vi "Read Elevator Command.vi"(6 "Reset Idle State":bool, 8 "Button Cluster":T3, 9 "Axes":dbl[](array[numeric]), 10 "Driver Buttons":bool[](array[boolean]), 11 "Call Context":T1) -> (0 "Idle Mode":T2, 3 "Command":T4)   [LabVIEW 2014]
uses:
  Elevator Command.ctl
  Common Code/Elevator Idle Mode.ctl
  Real-Life Controls/Button Cluster.ctl
  <vilib>/Rock Robotics/WPI/DriverStation/WPI_DriverStationDerivedRobotMode.ctl
  Common Code/Elevator State.ctl
  Common Code/Change Detect.vi
  Common Code/Change Detect Boolean.vi
  Robot Global Data.vi
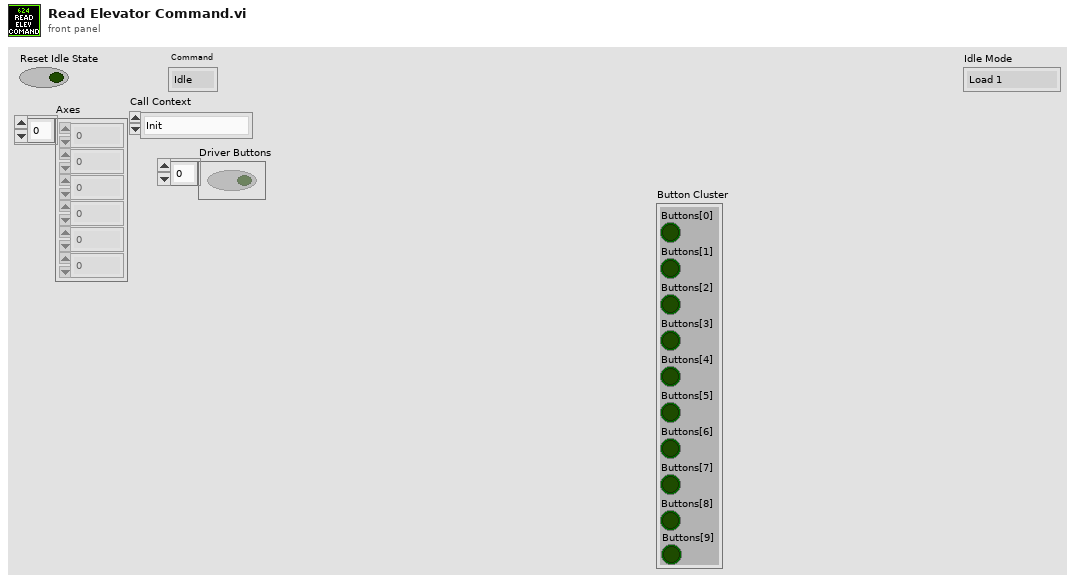
[diagram p1: front panel]
types:
  T1 = typedef "WPI_DriverStationDerivedRobotMode.ctl" = enum16{"Init", "Execute", "Stop"}
  T2 = typedef "Elevator Idle Mode.ctl" = enum16{"Load 1", "Load 2", "Load 3", "Load Can", "Untip Can", "Step Load", "Drop Stack", "Raw Height"}
  T3 = typedef "Button Cluster.ctl" = cluster{"Buttons[0]":bool, "Buttons[1]":bool, "Buttons[2]":bool, "Buttons[3]":bool, "Buttons[4]":bool, "Buttons[5]":bool, "Buttons[6]":bool, "Buttons[7]":bool, "Buttons[8]":bool, "Buttons[9]":bool}
  T4 = typedef "Elevator Command.ctl" = enum16{"Idle", "Load 1", "Load 2", "Load 3", "Drop Stack", "Eject Stack", "Untip Trashcan", "Load Trashcan", "HP Load", "HP Score"}
  T5 = typedef "Elevator State.ctl" = enum16{"Idle", "Goto Load Position", "Wait for Load", "Load Drop", "Load Lift", "Drop Stack", "Goto Eject Position", "Eject ", "Raise Trashcan", "Open Stabilizer", "Untip Drop", "Untip Wait", "Untip Lift", "Abort Load", "HP Load Wait", "HP Load Drop", "HP Load Lift", "HP Load Abort", "Close Stabilizer", "HP Load Unfinish", "HP Load Score", "HP Load Finish", "HP Goto Finish Down", "HP Goto Finish Up", "Full"}
  T6 = typedef "Elevator Status.ctl" = cluster{"Height":dbl, "Enc Value":dbl, "Limit Override":bool, "Mode":T7, "High IR":bool, "Motor Out":dbl, "Ping Detect":bool, "Auto Elevator Indicators":T8, "Master Current":dbl, "Slave Current":dbl, "High Current":bool, "Current Tripped":bool, "Top Limit":bool, "Bottom Limit":bool, "Eject Piston":bool, "Stabilizer":bool, "Finger":bool, "Finger Height":dbl, "Finger Raw":dbl, "Finger at Bottom":bool}
  T7 = typedef "Elevator Mode.ctl" = enum16{"Manual", "Safe", "Auto"}
  T8 = typedef "Auto Elevator Indicators.ctl" = cluster{"Target Out":dbl, "Storing Trashcan?":bool, "State":T5, "In Range":bool, "Store Can Command":bool, "HP Load":bool}
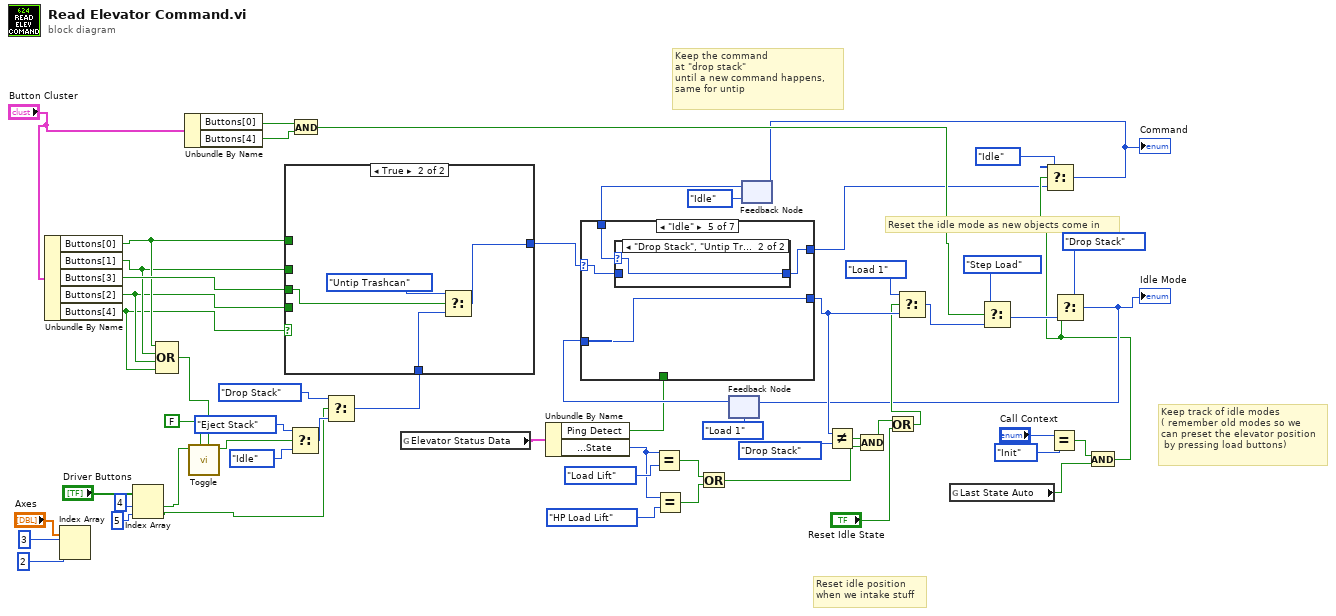
[diagram p0: block diagram]
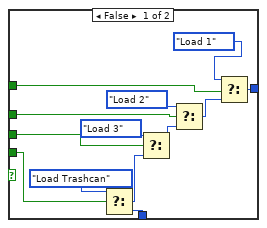
[diagram p2: hidden frame]
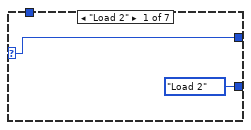
[diagram p3: hidden frame]
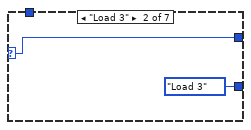
[diagram p4: hidden frame]
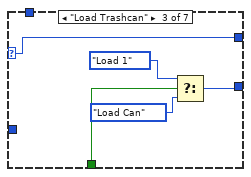
[diagram p5: hidden frame]
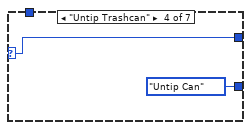
[diagram p6: hidden frame]
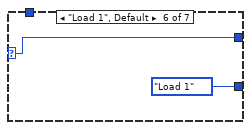
[diagram p8: hidden frame]
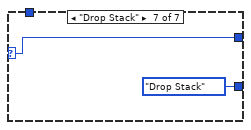
[diagram p9: hidden frame]
diagram:
  # "Keep the command\nat \"drop stack\"\nuntil a new command happens,\nsame for untip"
  # "Reset idle position\nwhen we intake stuff"
  # "Keep track of idle modes\n( remember old modes so we\ncan preset the elevator position\n by pressing load buttons)"
  # "Reset the idle mode as new objects come in"
  n1 = Unbundle By Name("Button Cluster") -> ("Buttons[0]"=w19:bool, "Buttons[1]"=w18:bool, "Buttons[3]"=w32:bool, "Buttons[2]"=w17:bool, "Buttons[4]"=w16:bool)
  n2 = Index Array(array="Axes", index #1=3 ("index"), index #2=2 ("index")) -> ()  [unwired: 2 out]
  n3 = Index Array(array="Driver Buttons", index #1=4 ("index"), index #2=5 ("index")) -> (element #1=w10:bool, element #2=w6:bool)
  n4 = Compound Arithmetic op=OR(w19, w18, w17, w16) -> (w15:bool)
  n5 = Unbundle By Name("Button Cluster") -> ("Buttons[0]"=w44:bool, "Buttons[4]"=w43:bool)
  n6 = call "Toggle.vi"("Reinit?"=w15, "Initial Value"=FALSE, "In"=w10) -> ("Toggled"=w20:bool)  [unwired: 8 in]
  n7 = Select(t=Elevator_Command."Eject Stack", s=w20, f=Elevator_Command."Idle" ("t")) -> (s? t:f=w56:T4)
  n8 = And(x=w44, y=w43) -> (x .and. y?=w42:bool)
  n9 = Select(t=Elevator_Command."Drop Stack", s=w6, f=w56) -> (s? t:f=w33:T4)
  n10 = case shown="True" w16 {
    tunnel: w33 -> [w64 w74]
    tunnel: [w63 w73] -> w49
    tunnel: w19 -> [w62 _]
    tunnel: w18 -> [w61 _]
    tunnel: w32 -> [w60 w72]
    tunnel: w17 -> [w59 _]
    frame False {
      n11 = Select(t=Elevator_Command."Load Trashcan", s=w59, f=w64) -> (s? t:f=w70:T4)
      n12 = Select(t=Elevator_Command."Load 3", s=w60, f=w70) -> (s? t:f=w66:T4)
      n13 = Select(t=Elevator_Command."Load 2", s=w61, f=w66) -> (s? t:f=w65:T4)
      n14 = Select(t=Elevator_Command."Load 1", s=w62, f=w65) -> (s? t:f=w63:T4)
    }
    frame True {
      n15 = Select(t=Elevator_Command."Untip Trashcan", s=w72, f=w74) -> (s? t:f=w73:T4)
    }
  }
  n16 = global read "Robot Global Data.vi" "Elevator Status Data"() -> (w31:T6)
  n17 = Unbundle By Name(w31) -> ("Ping Detect"=w21:bool, "Auto Elevator Indicators.State"=w28:T5)
  n18 = Equal?(x=w28, y=Elevator_State."Load Lift") -> (x = y?=w27:bool)
  n19 = Equal?(x=w28, y=Elevator_State."HP Load Lift") -> (x = y?=w25:bool)
  n20 = Or(x=w27, y=w25) -> (x .or. y?=w26:bool)
  n21 = feedback #1(Elevator_Idle_Mode."Load 1" ("Idle Mode")) -> (w48:T2)
  n22 = feedback #2(Elevator_Command."Idle" ("t")) -> (w36:T4)
  n23 = case shown="\"Idle\"" w49 {
    selector: w49 -> [w76 w78 w84 w85 w88 w93 w95]
    tunnel: [Elevator_Idle_Mode."Load 2" ("Idle Mode") Elevator_Idle_Mode."Load 3" ("Idle Mode") w80 Elevator_Idle_Mode."Untip Can" ("Idle Mode") w90 Elevator_Idle_Mode."Load 1" ("Idle Mode") Elevator_Idle_Mode."Drop Stack" ("Idle Mode")] -> w37
    tunnel: w48 -> [_ _ _ _ w90 _ _]
    tunnel: [w76 w78 w84 w85 w87 w93 w95] -> w2
    tunnel: w36 -> [_ _ _ _ w89 _ _]
    tunnel: w21 -> [_ _ w83 _ _ _ _]
    frame "Load 2" {
    }
    frame "Load 3" {
    }
    frame "Load Trashcan" {
      n24 = Select(t=Elevator_Idle_Mode."Load 1" ("Idle Mode"), s=w83, f=Elevator_Idle_Mode."Load Can" ("Idle Mode")) -> (s? t:f=w80:T2)
    }
    frame "Untip Trashcan" {
    }
    frame "Idle" {
      n25 = case shown="\"Drop Stack\", \"Untip Trashcan\"" w89 {
        selector: w89 -> [_ w92]
        tunnel: w88 -> [w91 _]
        tunnel: [w91 w92] -> w87
        frame "Idle", Default {
        }
        frame "Drop Stack", "Untip Trashcan" {
        }
      }
    }
    frame "Load 1", Default {
    }
    frame "Drop Stack" {
    }
  }
  n26 = Not Equal?(x=w37, y=Elevator_Idle_Mode."Drop Stack") -> (x != y?=w38:bool)
  n27 = Compound Arithmetic op=AND(w38, w26) -> (w23:bool)
  n28 = Or(x=w23, y="Reset Idle State") -> (x .or. y?=w22:bool)
  n29 = Select(t=Elevator_Idle_Mode."Load 1", s=w22, f=w37) -> (s? t:f=w41:T2)
  n30 = global read "Robot Global Data.vi" "Last State Auto"() -> (w11:bool)
  n31 = Select(t=Elevator_Idle_Mode."Step Load", s=w42, f=w41) -> (s? t:f=w9:T2)
  n32 = Equal?(x="Call Context", y=WPI_DriverStationDerivedRobotMode."Init") -> (x = y?=w12:bool)
  n33 = And(x=w12, y=w11) -> (x .and. y?=w4:bool)
  n34 = Select(t=Elevator_Command."Idle", s=w4, f=w2) -> (s? t:f=w1:T4)
  "Command" <- w1
  n35 = feedback-in #2(w1) -> ()
  n36 = Select(t=Elevator_Idle_Mode."Drop Stack", s=w4, f=w9) -> (s? t:f=w7:T2)
  "Idle Mode" <- w7
  n37 = feedback-in #1(w7) -> ()
